vi "DSF.Engine.Memory.ObjectPool.Bundle.Get Index.vi"(8 "error in (no error)":errorcluster, 11 "ObjectPool Bundle in":refnum<class "DSF.Engine.Memory.ObjectPool.Bundle.lvclass">) -> (0 "error out":errorcluster, 2 "index":i32, 3 "ObjectPool Bundle out":refnum<class "DSF.Engine.Memory.ObjectPool.Bundle.lvclass">)   [LabVIEW 2016, in "DSF.Engine.lvlib" / "DSF.Engine.Memory.ObjectPool.Bundle.lvclass"]
uses:
  DSF.Engine.Memory.ObjectPool.Bundle.lvclass
  DSF.Engine.Memory.ObjectPool.Bundle.lvclass/DSF.Engine.Memory.ObjectPool.Bundle.ctl
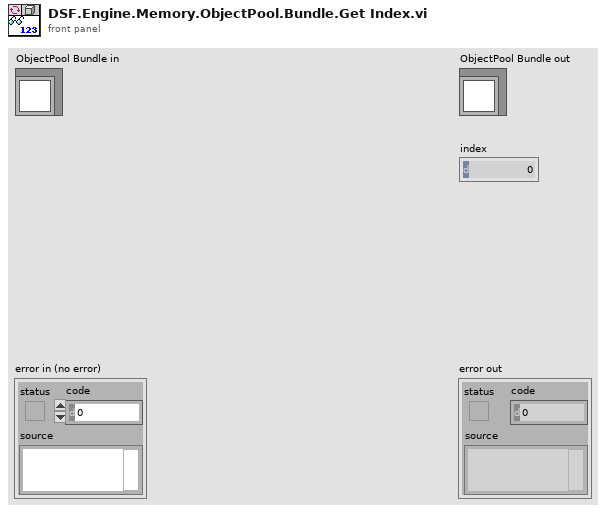
[diagram p1: front panel]
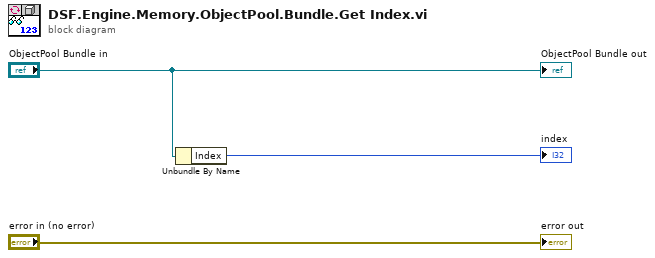
[diagram p0: block diagram]
diagram:
  n1 = Unbundle By Name("ObjectPool Bundle in") -> ("Index"=→"index":i32)
  "error out" <- "error in (no error)"
  "ObjectPool Bundle out" <- "ObjectPool Bundle in"
